vi "Event Handler - Sequence List - Key Up.vi"(4 "User Parameter":T1, 5 "Event Data":cluster{"keyCode":i16, "shift":i16}, 6 "Control Ref":refnum<k7>, 7 "Event Common Data":T2) -> ()   [LabVIEW 2021, in "Seq Edit Quick Drop.lvlib"]
uses:
  Seq Edit Quick Drop.lvlib
  Event Data.ctl
  Connection Type.ctl
  Event Response.ctl
  Message.ctl
  Command.ctl
  Key Codes Constants.vi
  Settings.vi
  <vilib>/Utility/SystemLogging/NI_SystemLogging.lvlib
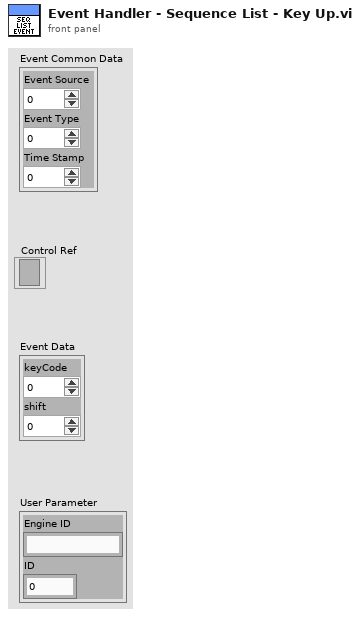
[diagram p1: front panel]
types:
  T1 = typedef "Seq Edit Quick Drop.lvlib/Event Data.ctl" = cluster{"Engine ID":string, "ID":i32}
  T2 = cluster{"Event Source":i32, "Event Type":u32, "Time Stamp":u32}
  T3 = typedef "Seq Edit Quick Drop.lvlib/Event Response.ctl" = cluster{"Connection Type":T4, "ID":i32}
  T4 = typedef "Seq Edit Quick Drop.lvlib/Connection Type.ctl" = enum16{"SequenceView", "SequenceList", "VariablesView"}
  T5 = cluster{"Key":string, "Modifiers":cluster{"SHIFT":bool, "CONTROL":bool, "ALT":bool}}
  T6 = cluster{"SHIFT":bool, "CONTROL":bool, "ALT":bool}
  T7 = typedef "Seq Edit Quick Drop.lvlib/Message.ctl" = cluster{"cmd":T8, "data":variant}
  T8 = typedef "Seq Edit Quick Drop.lvlib/Command.ctl" = enum16{"Init", "Get Application Manager", "Shortcut Activated", "Display Tools", "Tool Selected", "Timeout", "Error", "Close"}
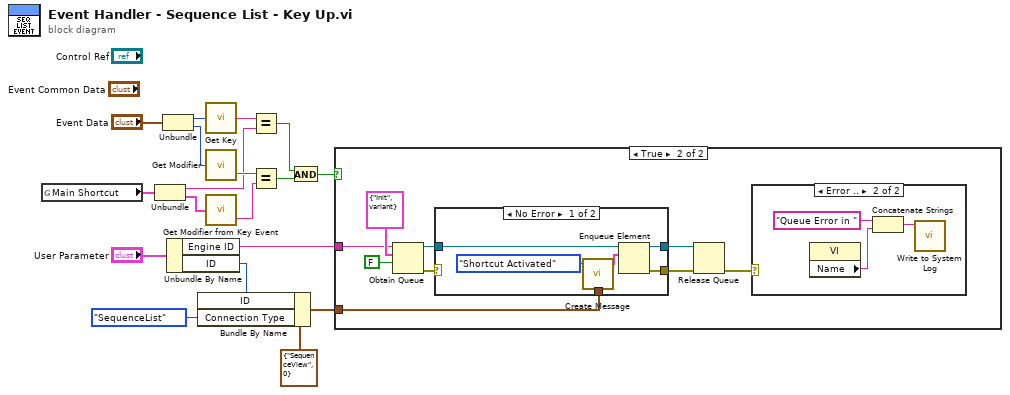
[diagram p0: block diagram]
diagram:
  n1 = global read "Settings.vi" "Main Shortcut"() -> (w12:T5)
  n2 = Unbundle(w12) -> ("Key"=w11:string, "Modifiers"=w2:T6)
  n3 = Unbundle("Event Data") -> ("keyCode"=w18:i16, "shift"=w17:i16)
  n4 = Unbundle By Name("User Parameter") -> ("Engine ID"=w9:string, "ID"=w6:i32)
  n5 = Bundle By Name(cluster=T3 {"Connection Type"=enum."SequenceView", "ID"=0} ("Event Response"), "ID"=w6, "Connection Type"=Connection_Type."SequenceList") -> (w5:T3)
  n6 = call "Get Key.vi"("Key Code"=w18) -> ("Key"=w16:string)
  n7 = call "Get Modifier.vi"("Modifier Code"=w17) -> ("Modifiers Concatenated"=w15:string)  [unwired: 1 out]
  n8 = call "Get Modifier from Key Event.vi"("Modifiers"=w2) -> ("Modifiers Concatenated"=w1:string)  [unwired: 1 out]
  n9 = Equal?(x=w16, y=w11) -> (x = y?=w14:bool)
  n10 = Equal?(x=w15, y=w1) -> (x = y?=w13:bool)
  n11 = And(x=w14, y=w13) -> (x .and. y?=w10:bool)
  n12 = case shown="True" w10 {
    tunnel: w9 -> [_ w23]
    tunnel: w5 -> [_ w21]
    frame False {
    }
    frame True {
      n13 = Obtain Queue(name (unnamed)=w23, element data type=T7 {"cmd"=enum."Init", "data"=variant} ("msg"), create if not found? (T)=FALSE) -> (queue out=w25:refnum<queue>, error out=w24:errorcluster)  [unwired: 2 in, 1 out]
      n14 = case shown="No Error" w24 {
        selector: w24 -> [_ w38]
        tunnel: w25 -> [w34 w37]
        tunnel: [w33 w38] -> w22
        tunnel: w21 -> [w32 _]
        tunnel: [w31 w37] -> w19
        frame No Error {
          n15 = call "Create Message.vi"("cmd"=Command."Shortcut Activated", "data"=w32) -> ("msg"=w35:T7)  [unwired: 2 in]
          n16 = Enqueue Element(queue=w34, element=w35) -> (queue out=w31:refnum<queue>, error out=w33:errorcluster)  [unwired: 2 in, 1 out]
        }
        frame Error {
        }
      }
      n17 = Release Queue(queue=w19, error in (no error)=w22) -> (error out=w20:errorcluster)  [unwired: 1 in, 2 out]
      n18 = case shown="Error .." w20 {
        frame No Error {
        }
        frame Error {
          n19 = property class="VI"() -> ("Name"=w29:string)  [unwired: 2 in, 2 out]
          n20 = Concatenate Strings("Queue Error in " ("string"), w29) -> (w28:string)
          n21 = call <vilib>:"Write to System Log.vi"("message"=w28) -> ()  [unwired: 10 in, 1 out]
        }
      }
    }
  }
